vi "brown.vi"() -> (1 "brown":dbl, 2 "brown/2":dbl)   [LabVIEW 2014]
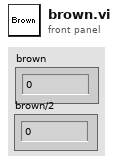
[diagram p1: front panel]
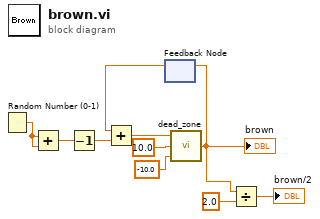
[diagram p0: block diagram]
diagram:
  n1 = Random Number (0-1)() -> (number: 0 to 1=w10:dbl)
  n2 = Add(x=w10, y=w10) -> (x+y=w9:dbl)
  n3 = Decrement(x=w9) -> (x-1=w8:dbl)
  n4 = feedback #1() -> (w1:dbl)  [unwired: 1 in]
  n5 = Add(x=w1, y=w8) -> (x+y=w7:dbl)
  n6 = call "dead_zone.vi"("min"=-10.0, "max"=10.0, "number in"=w7) -> ("number out"=w2:dbl)
  "brown" <- w2
  n7 = feedback-in #1(w2) -> ()
  n8 = Divide(x=w2, y=2.0) -> (x/y=→"brown/2":dbl)
